vi "Read Hardware Version.vi"(0 "Session Handle in":T1, 11 "error in (no error)":errorcluster) -> (4 "Session Handle out":T1, 6 "Hardware Version":string, 15 "error out":errorcluster)   [LabVIEW 2015, in "PAS.lvclass"]
uses:
  PAS.lvclass
  Typedefs/Session Handle.ctl
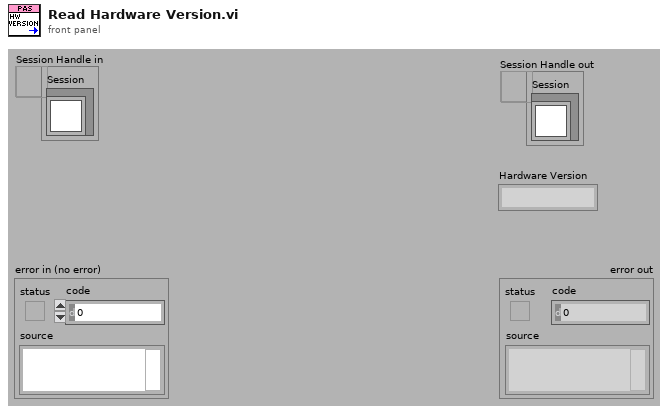
[diagram p1: front panel]
types:
  T1 = typedef "PAS.lvclass/Session Handle.ctl" = refnum<data-value>
  T2 = typedef "XNET Frame CAN.ctl" = cluster{"timestamp":timestamp, "payload":u8[], "identifier":u32, "type":T3, "extended?":bool, "echo?":bool}
  T3 = typedef "XNET Frame Type CAN.ctl" = u8
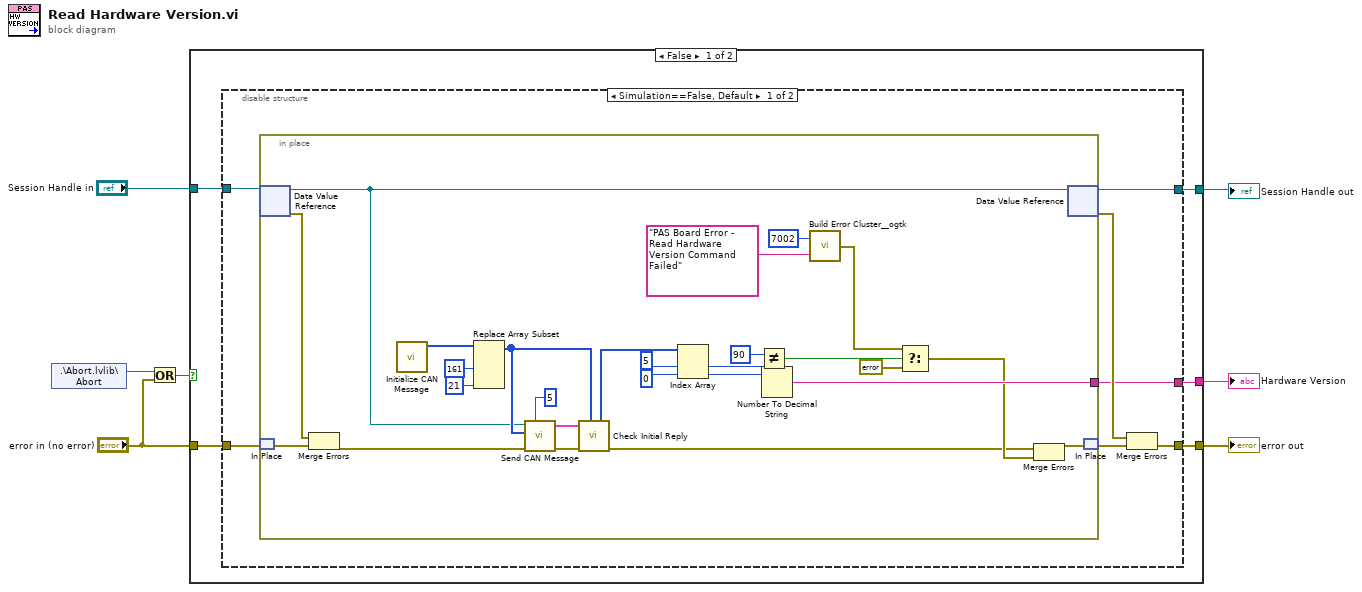
[diagram p0: block diagram]
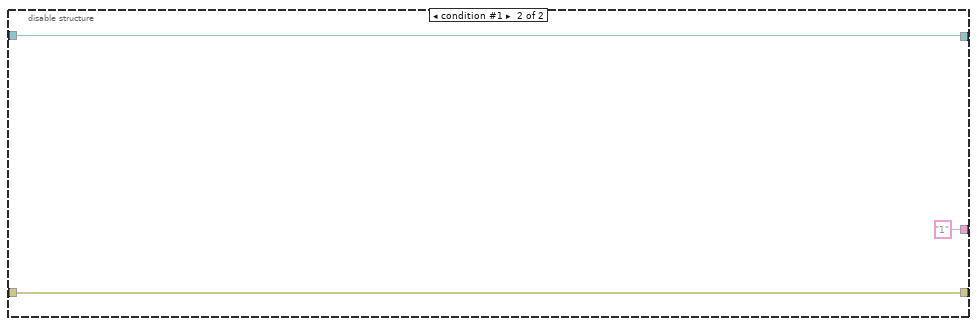
[diagram p2: hidden frame]
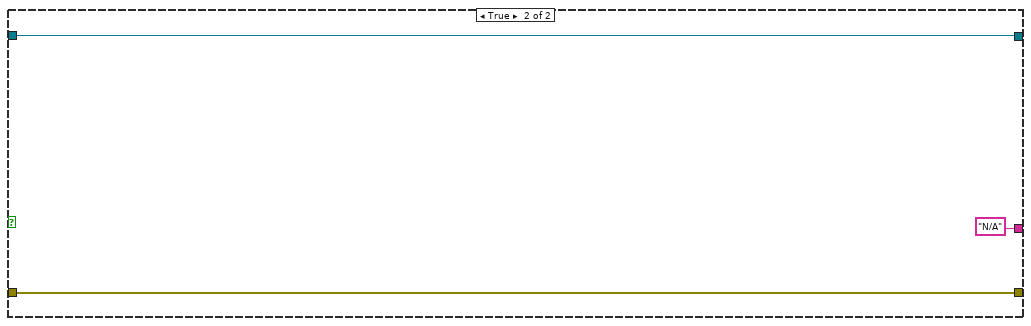
[diagram p3: hidden frame]
diagram:
  n1 = shared-variable ".\\Abort.lvlib\\Abort"() -> (w4:bool)  [unwired: 1 in, 1 out]
  n2 = Or(x=w4, y="error in (no error)") -> (x .or. y?=w2:bool)
  n3 = case shown="False" w2 {
    tunnel: [w12 w51] -> w6
    tunnel: [w11 w50] -> w5
    tunnel: "Session Handle in" -> [w10 w51]
    tunnel: "error in (no error)" -> [w9 w50]
    tunnel: [w8 "N/A"] -> w1
    frame False {
      n4 = disable-structure shown="Simulation==False, Default" {
        disable-tunnel: [w19 w48] -> w12
        disable-tunnel: [w16 w47] -> w11
        disable-tunnel: w10 -> [w15 w48]
        disable-tunnel: w9 -> [w14 w47]
        disable-tunnel: [w13 "1"] -> w8
        frame condition #0 (active) {
          n5 = in-place {
            in-place-border: [w23] -> w13
            n6 = in-place-dvr #1(w15) -> (w36:refnum<class "PAS.lvclass">, w40:errorcluster)
            n7 = in-place-match #2(w14) -> (w39:errorcluster)
            n8 = Merge Errors(w40, w39) -> (w38:errorcluster)
            n9 = call "Initialize CAN Message.vi"() -> ("Initial Payload"=w42:u8[])  [unwired: 11 in]
            n10 = Replace Array Subset(array=w42, new element #1=u8 161 ("new element/subarray"), new element #2=u8 21 ("new element/subarray")) -> (w37:u8[])  [unwired: 2 in]
            n11 = call "Send CAN Message.vi"("Number of Retries"=5, "error in (no error)"=w38, "payload"=w37, "Gas In"=w36) -> ("error out"=w21:errorcluster, "Reply"=w34:T2[])  [unwired: 5 in, 1 out]
            n12 = call "Check Initial Reply.vi"("Write Message"=w37, "error in (no error)"=w21, "Reply"=w34) -> ("error out"=w20:errorcluster, "Data Packet"=w41:u8[])  [unwired: 5 in, 2 out]
            n13 = Index Array(array=w41, index #1=5 ("index"), index #2=0 ("index")) -> (element #1=w28:u8, element #2=w25:u8)
            n14 = Not Equal?(x=u8 90 ("new element/subarray"), y=w28) -> (x != y?=w26:bool)
            n15 = Number To Decimal String(number=w25) -> (decimal integer string=w23:string)  [unwired: 1 in]
            n16 = call <userlib>:"Build Error Cluster__ogtk.vi"("String to Prepend to source (\"\")"="PAS Board Error - Read Hardware Version Command Failed" ("string"), "code"=7002) -> ("error out"=w31:errorcluster)
            n17 = Select(t=w31, s=w26, f=errorcluster {"status"=FALSE, "code"=0, "source"=""}) -> (s? t:f=w22:errorcluster)
            n18 = Merge Errors(w20, w22) -> (w43:errorcluster)
            n19 = in-place-dvr #1(w36) -> (w19:T1, w17:errorcluster)
            n20 = in-place-match #2(w43) -> (w18:errorcluster)
          }
          n21 = Merge Errors(w17, w18) -> (w16:errorcluster)
        }
        frame condition #1 {
        }
      }
    }
    frame True {
    }
  }
  "Session Handle out" <- w6
  "error out" <- w5
  "Hardware Version" <- w1
